vi "3DDraw.vi"(11 "Beta/gamma":T1(array[cluster])=[{"Color"=14090460, "Length"=1.0, "Base position"={"X"=0.5, "Y"=0.0}, "Joint Angle"=30.0}, {"Color"=14090460, "Length"=1.0, "Base position"={"X"=-0.5, "Y"=0.0}, "Joint Angle"=150.0}, {"Color"=12171705, "Length"=1.3, "Base position"={"X"=1.0, "Y"=1.0}, "Joint Angle"=120.0}, {"Color"=12171705, "Length"=1.3, "Base position"={"X"=-1.0, "Y"=1.0}, "Joint Angle"=30.0}]) -> (3 "3D Picture":refnum<vi>(3d-picture))   [LabVIEW 2022 SP3]
uses:
  <vilib>/picture/3D Picture Control/Object/Create Object (name).vi
  <vilib>/picture/3D Picture Control/NI_3D Picture Control.lvlib
panel:
  in  "beam height":dbl=0.1
  in  "beam width":dbl=0.1
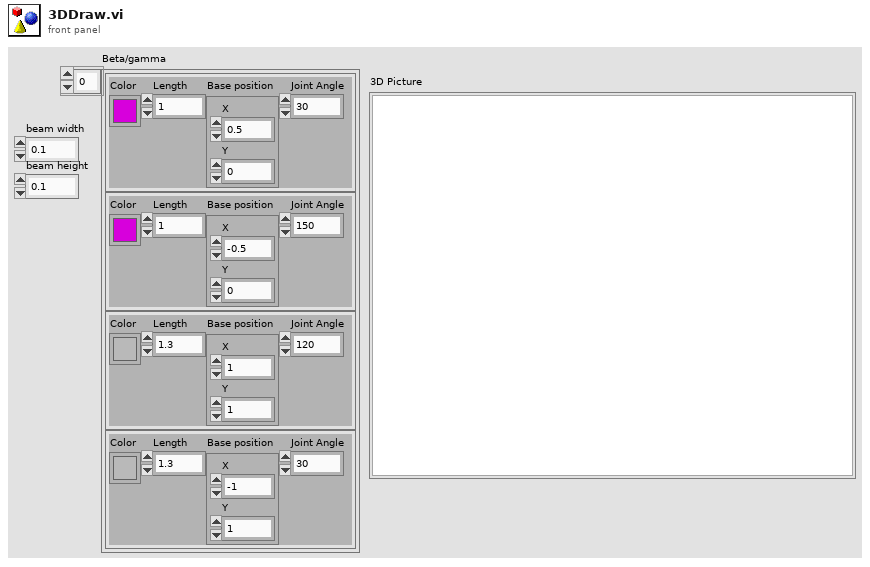
[diagram p1: front panel]
types:
  T1 = cluster{"Color":u32, "Length":dbl, "Base position":cluster{"X":dbl, "Y":dbl}, "Joint Angle":dbl}[]
  T2 = cluster{"output cluster":cluster{dbl, dbl, dbl}, "Joint Angle":dbl}
  T3 = cluster{"Color":u32, "Length":dbl, cluster{"Length":dbl, dbl, dbl}, cluster{"output cluster":cluster{dbl, dbl, dbl}, "Joint Angle":dbl}, cluster{"X":dbl, "Y":dbl, dbl}}
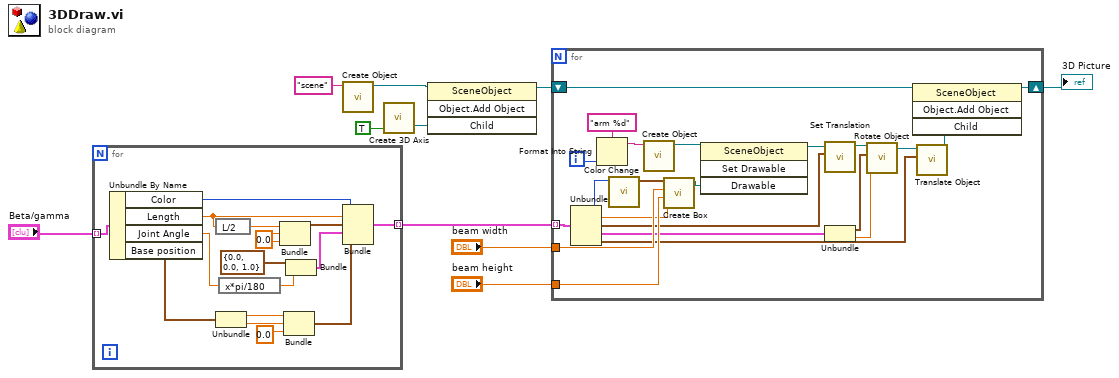
[diagram p0: block diagram]
diagram:
  n1 = for {
    tunnel: "Beta/gamma" -> [w26] mode=indexing
    tunnel: [w11] -> w1 mode=indexing
    w24 = 0.0
    n2 = Unbundle By Name(w26) -> ("Color"=w25:u32, "Length"=w22:dbl, "Joint Angle"=w18:dbl, "Base position"=w16:cluster{"X":dbl, "Y":dbl})
    n3 = expression code="L/2"(w22) -> (w23:dbl)
    n4 = Unbundle(w16) -> ("X"=w15:dbl, "Y"=w14:dbl)
    n5 = expression code="x*pi/180"(w18) -> (w20:dbl)
    n6 = Bundle("Length"=w23, w24, w24) -> (w21:cluster{"Length":dbl, dbl, dbl})  [unwired: 1 in]
    n7 = Bundle("X"=w15, "Y"=w14, 0.0) -> (w12:cluster{"X":dbl, "Y":dbl, dbl})  [unwired: 1 in]
    n8 = Bundle("output cluster"=cluster{dbl, dbl, dbl} {0.0, 0.0, 1.0}, "Joint Angle"=w20) -> (w17:T2)  [unwired: 1 in]
    n9 = Bundle("Color"=w25, "Length"=w22, w21, w17, w12) -> (w11:T3)  [unwired: 1 in]
  }
  n10 = call-poly <vilib>:"Create Object.vi"("Name"="scene") -> ("Scene:New Object"=w5:refnum<vi>)  [unwired: 9 in, 1 out]
  n11 = call <vilib>:"Create 3D Axis.vi"("Axis label?"=TRUE) -> ("New Object Refnum"=w6:refnum<vi>)  [unwired: 9 in, 1 out]
  n12 = invoke class="SceneObject" method="Object.Add Object"(reference=w5, "Child"=w6) -> (reference out=w4:refnum<vi>)  [unwired: 2 in, 3 out]
  n13 = for {
    shift-right: [w45] -> w9
    shift-left: w4 -> [w46]
    tunnel: "beam width" -> [w40]
    tunnel: "beam height" -> [w39]
    tunnel: w1 -> [w38] mode=indexing
    i -> [w43]
    n14 = Unbundle(w38) -> ("Color"=w37:u32, "Length"=w36:dbl, w35:cluster{"Length":dbl, dbl, dbl}, w34:T2, w29:cluster{"X":dbl, "Y":dbl, dbl})
    n15 = Format Into String(format string="arm %d" ("Name"), w43) -> (resulting string=w42:string)  [unwired: 2 in, 1 out]
    n16 = call <vilib>:"Color Change.vi"("Color"=w37) -> ("RGBA"=w41:cluster{"R":sgl, "G":sgl, "B":sgl, "A":sgl})  [unwired: 10 in]
    n17 = call-poly <vilib>:"Create Object.vi"("Name"=w42) -> ("Scene:New Object"=w48:refnum<vi>)  [unwired: 9 in, 1 out]
    n18 = call <vilib>:"Create Box.vi"("Color"=w41, "Length Z"=w39, "Length Y"=w40, "Length X"=w36) -> ("New Box Refnum"=w47:refnum<vi>)  [unwired: 6 in, 1 out]
    n19 = invoke class="SceneObject" method="Set Drawable"(reference=w48, "Drawable"=w47) -> (reference out=w32:refnum<vi>)  [unwired: 2 in, 3 out]
    n20 = call <vilib>:"Set Translation.vi"("Translation"=w35, "Scene Object"=w32) -> ("Translated Object"=w31:refnum<vi>)  [unwired: 8 in, 1 out]
    n21 = Unbundle(w34) -> ("output cluster"=w33:cluster{dbl, dbl, dbl}, "Joint Angle"=w27:dbl)
    n22 = call <vilib>:"Rotate Object.vi"("Angle"=w27, "Axis"=w33, "Scene.Object In"=w31) -> ("Scene.Object Out"=w30:refnum<vi>)  [unwired: 7 in, 1 out]
    n23 = call <vilib>:"Translate Object.vi"("Translation"=w29, "Scene.Object In"=w30) -> ("Scene.Object Out"=w28:refnum<vi>)  [unwired: 8 in, 1 out]
    n24 = invoke class="SceneObject" method="Object.Add Object"(reference=w46, "Child"=w28) -> (reference out=w45:refnum<vi>)  [unwired: 2 in, 3 out]
  }
  "3D Picture" <- w9
